vi "Set Data Out.vi"(8 "error in (no error)":errorcluster, 11 "DataOut":T1) -> (0 "error out":errorcluster)   [LabVIEW 2017]
uses:
  TypeDefs/dataOut.ctl
  FGVs/TypeDefs/DataFGVControl.ctl
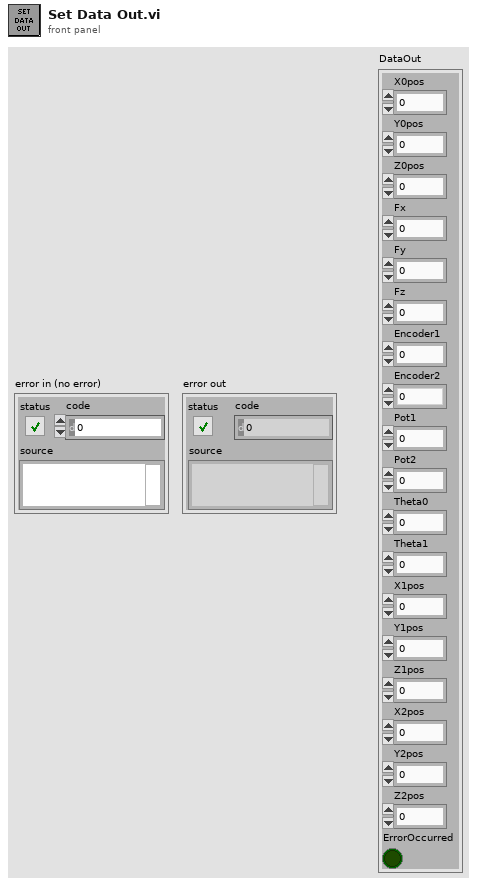
[diagram p1: front panel]
types:
  T1 = typedef "dataOut.ctl" = cluster{"X0pos":dbl, "Y0pos":dbl, "Z0pos":dbl, "Fx":dbl, "Fy":dbl, "Fz":dbl, "Encoder1":i32, "Encoder2":i32, "Pot1":dbl, "Pot2":dbl, "Theta0":dbl, "Theta1":dbl, "X1pos":dbl, "Y1pos":dbl, "Z1pos":dbl, "X2pos":dbl, "Y2pos":dbl, "Z2pos":dbl, "ErrorOccurred":bool}
  T2 = typedef "DataFGVControl.ctl" = enum16{"Set Data", "Get Data"}
  T3 = typedef "allData.ctl" = cluster{"DataOut":T1, "DataIn":T4}
  T4 = typedef "dataIn.ctl" = cluster{"Xtarget":dbl, "Ytarget":dbl, "Ztarget":dbl, "X_Attractor 1":dbl, "Y_Attractor 1":dbl, "Z_Attractor 1":dbl, "X_Attractor 2":dbl, "Y_Attractor 2":dbl, "Z_Attractor 2":dbl, "Traj Flag":bool, "DeadZone":dbl, "Assistance":bool, "Shutdown?":bool, "AssistanceLevel":dbl}
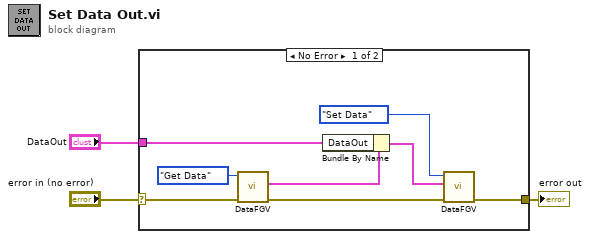
[diagram p0: block diagram]
diagram:
  n1 = case shown="No Error" "error in (no error)" {
    selector: "error in (no error)" -> [w11 w12]
    tunnel: [w8 w12] -> w2
    tunnel: "DataOut" -> [w6 _]
    frame No Error {
      n2 = call "DataFGV.vi"("error in (no error)"=w11, "Command"=DataFGVControl."Get Data") -> ("error out"=w9:errorcluster, "AllData out"=w7:T3)  [unwired: 8 in]
      n3 = Bundle By Name(cluster=w7, "DataOut"=w6) -> (w5:T3)
      n4 = call "DataFGV.vi"("error in (no error)"=w9, "AllData in"=w5, "Command"=DataFGVControl."Set Data") -> ("error out"=w8:errorcluster)  [unwired: 7 in, 1 out]
    }
    frame Error {
    }
  }
  "error out" <- w2
